vi "Get Module Running State.vi"() -> (3 "Module Running State":T1)   [LabVIEW 2015, in "Device Under Test_Cloneable_DQMH.lvlib"]
doc: "Determine if the cloneable module is not running, running as cloneable, or running as singleton.\n____\nDelacor QMH Thermal Chamber Examples 4.0.0.21\nCopyright (c) 2018, Delacor"
uses:
  Device Under Test_Cloneable_DQMH.lvlib
  Module Running State--enum.ctl
  Clone Registration/Clone Registration.lvlib
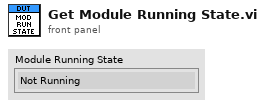
[diagram p1: front panel]
types:
  T1 = typedef "Device Under Test_Cloneable_DQMH.lvlib/Module Running State--enum.ctl" = enum16{"Not Running", "Running as Cloneable", "Running as Singleton"}
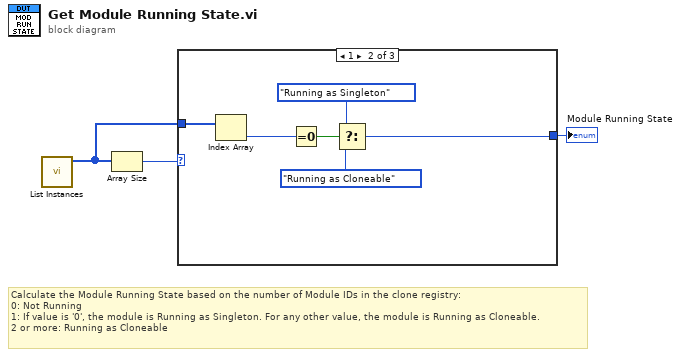
[diagram p0: block diagram]
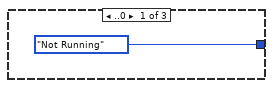
[diagram p2: hidden frame]
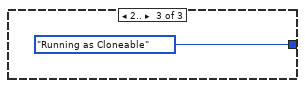
[diagram p3: hidden frame]
diagram:
  # "Calculate the Module Running State based on the number of Module IDs in the clone registry:\n0: Not Running\n1: If value is '0', the module is Running as Singleton. For any other value, the module is Running as Cloneable.\n2 or more: Running as Cloneable"
  n1 = call "List Instances.vi"() -> ("Module IDs"=w1:i32[])  [unwired: 7 in, 4 out]
  n2 = Array Size(array=w1) -> (size(s)=w3:i32)
  n3 = case shown="1" w3 {
    tunnel: [Module_Running_State--enum."Not Running" ("Module Running State") w5 Module_Running_State--enum."Running as Cloneable" ("Module Running State")] -> w2
    tunnel: w1 -> [_ w10 _]
    frame ..0 {
    }
    frame 1 {
      n4 = Index Array(array=w10) -> (element=w9:i32)  [unwired: 1 in]
      n5 = Equal To 0?(x=w9) -> (x = 0?=w8:bool)
      n6 = Select(t=Module_Running_State--enum."Running as Singleton" ("Module Running State"), s=w8, f=Module_Running_State--enum."Running as Cloneable" ("Module Running State")) -> (s? t:f=w5:T1)
    }
    frame 2.. {
    }
  }
  "Module Running State" <- w2
